vi "All Not Complex.vi"() -> (3 "Benchmark":cluster{i32[], dbl[]}[](graph))   [LabVIEW 2020]
doc: "Execute GEMM Process for different size on different Toolkits (Accelerator/Culab/CUDA/LabVIEW/G2CPU) and LabVIEW(CPU)."
panel:
  out "Accelerator DirectML":bool
  out "Accelerator CUDA":bool
  out "Culab":bool
  out "Accelerator TRT":bool
  out "LabVIEW":bool
  out "G2CPU":bool
  out "LabVIEW Toolkit Time":dbl
  out "G2CPU Time":dbl
  out "Accelerator CUDA Times":dbl[](array[numeric])
  out "Accelerator CUDA Time":dbl
  out "LabVIEW Times":dbl[](array[numeric])
  out "G2CPU Times":dbl[](array[numeric])
  out "Culab Times":dbl[](array[numeric])
  out "Accelerator TRT Times":dbl[](array[numeric])
  out "Culab Time":dbl
  out "Accelerator TRT Time":dbl
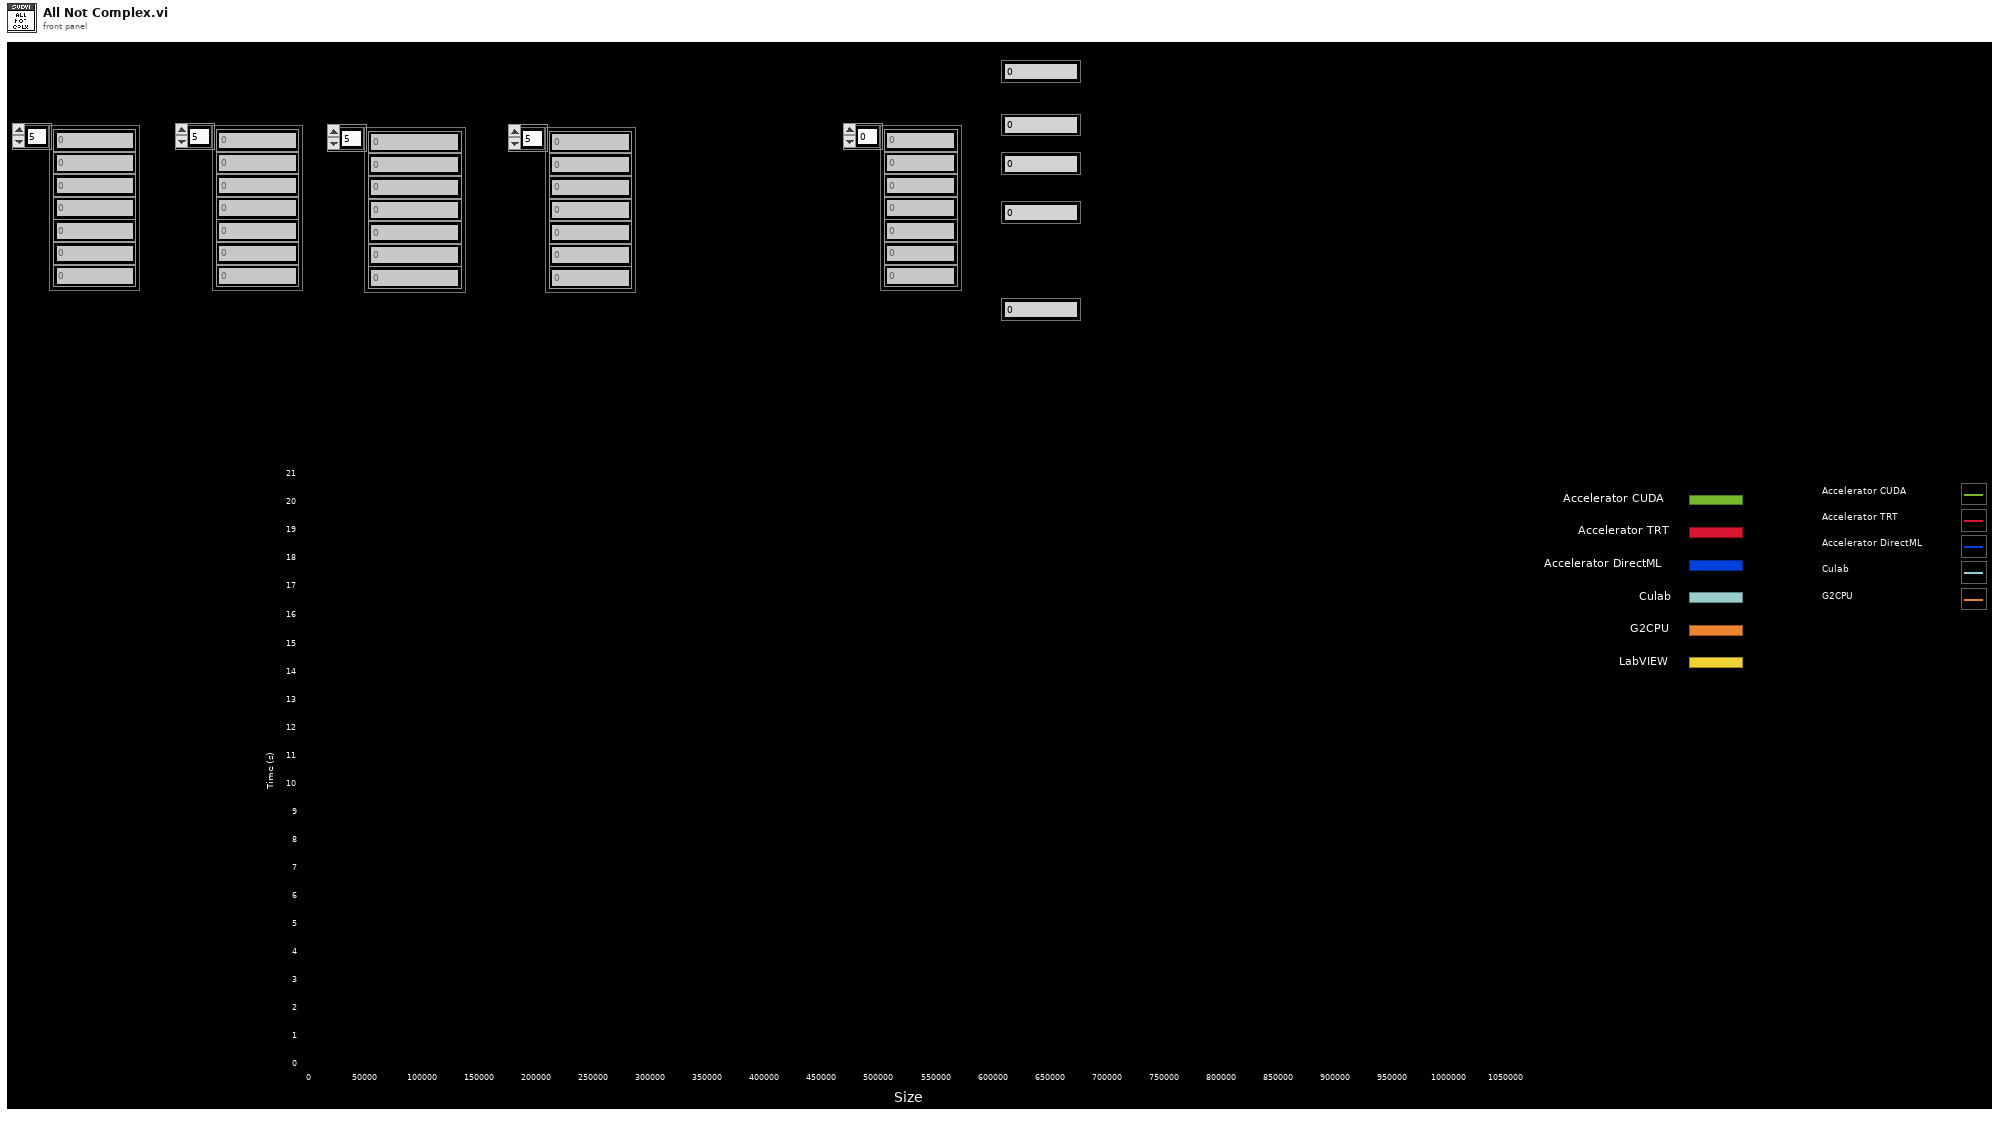
[diagram p1: front panel]
types:
  T1 = cluster{"intra_op_num_threads":i32, "inter_op_num_threads":i32, "execution_mode":enum16{"ORT_SEQUENTIAL", "ORT_PARALLEL"}, "deterministic_compute":bool, "graph_optimization_level":u16, "optimized_model_file_path":path, "profiling output dir":path}
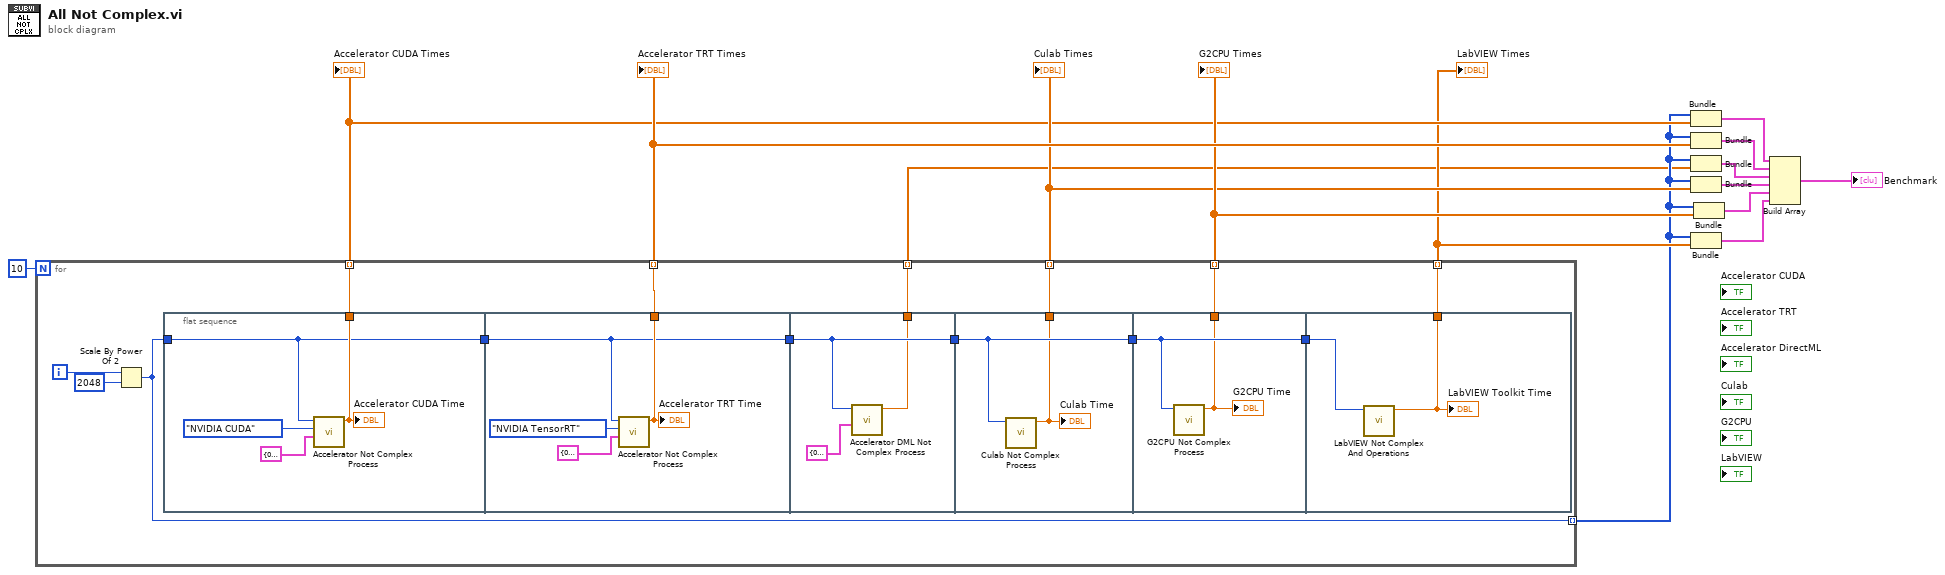
[diagram p0: block diagram]
diagram:
  n1 = for {
    N: 10 -> [_]
    tunnel: [w28] -> w14 mode=indexing
    tunnel: [w27] -> w12 mode=indexing
    tunnel: [w26] -> w13 mode=indexing
    tunnel: [w22] -> w2 mode=indexing
    tunnel: [w20] -> w7 mode=indexing
    tunnel: [w19] -> w6 mode=indexing
    tunnel: [w16] -> w1 mode=indexing
    i -> [w24]
    n2 = Scale By Power Of 2(n=w24, x=2048) -> (x*2^n=w22:i32)
    n3 = flat-sequence {
      tunnel: w22 -> [w30]
      tunnel: [w30] -> w21
      tunnel: [w33] -> w20
      tunnel: [w36] -> w18
      tunnel: [w37] -> w28
      tunnel: w21 -> [w36]
      tunnel: w18 -> [w40]
      tunnel: [w40] -> w17
      tunnel: [w38] -> w16
      tunnel: w17 -> [w42]
      tunnel: [w42] -> w29
      tunnel: [w41] -> w27
      tunnel: w29 -> [w44]
      tunnel: [w43] -> w26
      tunnel: [w44] -> w23
      tunnel: [w45] -> w19
      tunnel: w23 -> [w46]
      frame #0 {
        n4 = call "Accelerator Not Complex Process.vi"("Sessions Parameters"=T1 {"intra_op_num_threads"=0, "inter_op_num_threads"=0, "execution_mode"=enum."ORT_SEQUENTIAL", "deterministic_compute"=FALSE, "graph_optimization_level"=1, "optimized_model_file_path"=path "", "profiling output dir"=path ""}, "Execution Device"=enum16{"CPU", "NVIDIA CUDA", "NVIDIA TensorRT"}."NVIDIA CUDA", "X size"=w30) -> ("Accelerator Time"=w33:dbl)  [unwired: 8 in]
        "Accelerator CUDA Time" <- w33
      }
      frame #1 {
        n5 = call "Accelerator Not Complex Process.vi"("Sessions Parameters"=T1 {"intra_op_num_threads"=0, "inter_op_num_threads"=0, "execution_mode"=enum."ORT_SEQUENTIAL", "deterministic_compute"=FALSE, "graph_optimization_level"=1, "optimized_model_file_path"=path "", "profiling output dir"=path ""}, "Execution Device"=enum16{"CPU", "NVIDIA CUDA", "NVIDIA TensorRT"}."NVIDIA TensorRT", "X size"=w36) -> ("Accelerator Time"=w37:dbl)  [unwired: 8 in]
        "Accelerator TRT Time" <- w37
      }
      frame #2 {
        n6 = call "Accelerator DML Not Complex Process.vi"("Sessions Parameters"=T1 {"intra_op_num_threads"=0, "inter_op_num_threads"=0, "execution_mode"=enum."ORT_SEQUENTIAL", "deterministic_compute"=FALSE, "graph_optimization_level"=1, "optimized_model_file_path"=path "", "profiling output dir"=path ""}, "X size"=w40) -> ("Accelerator Time"=w38:dbl)  [unwired: 9 in]
      }
      frame #3 {
        n7 = call "Culab Not Complex Process.vi"("X size"=w42) -> ("Culab Time"=w41:dbl)  [unwired: 10 in]
        "Culab Time" <- w41
      }
      frame #4 {
        n8 = call "G2CPU Not Complex Process.vi"("X size"=w44) -> ("G2CPU Time"=w43:dbl)  [unwired: 10 in]
        "G2CPU Time" <- w43
      }
      frame #5 {
        n9 = call "LabVIEW Not Complex And Operations.vi"("X size"=w46) -> ("LabVIEW Time"=w45:dbl)  [unwired: 10 in]
        "LabVIEW Toolkit Time" <- w45
      }
    }
  }
  "Accelerator TRT Times" <- w14
  "Culab Times" <- w12
  "G2CPU Times" <- w13
  "LabVIEW Times" <- w6
  "Accelerator CUDA Times" <- w7
  n10 = Bundle(w2, w7) -> (w8:cluster{i32[], dbl[]})  [unwired: 1 in]
  n11 = Bundle(w2, w14) -> (w9:cluster{i32[], dbl[]})  [unwired: 1 in]
  n12 = Bundle(w2, w1) -> (w3:cluster{i32[], dbl[]})  [unwired: 1 in]
  n13 = Bundle(w2, w12) -> (w4:cluster{i32[], dbl[]})  [unwired: 1 in]
  n14 = Bundle(w2, w6) -> (w5:cluster{i32[], dbl[]})  [unwired: 1 in]
  n15 = Bundle(w2, w13) -> (w11:cluster{i32[], dbl[]})  [unwired: 1 in]
  n16 = Build Array(w8, w9, w3, w4, w11, w5) -> (→"Benchmark":cluster{i32[], dbl[]}[])
